vi "GetSingleAxisPos.vi"(6 "milliseconds to wait":u32=2, 8 "error in":errorcluster, 11 "Axis":T1={"System #"=0, "Axis ID"="", "Multiplier"=1.0}) -> (0 "error out":errorcluster, 3 "Position":dbl)   [LabVIEW 2011]
uses:
  PI_Axis.ctl
  PIAxisInfoGlobal.vi
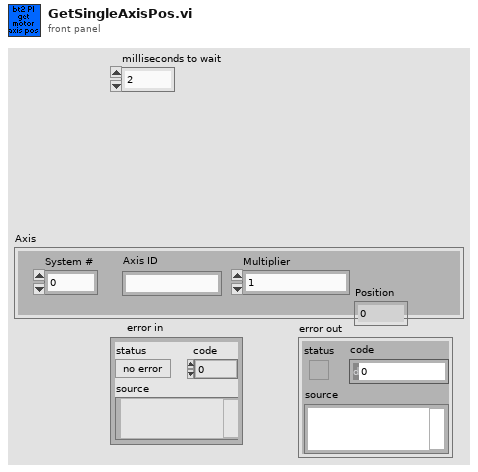
[diagram p1: front panel]
types:
  T1 = typedef "PI_Axis.ctl" = cluster{"System #":i32, "Axis ID":string, "Multiplier":dbl}
  T2 = typedef "GCS_Interface.ctl" = cluster{"MOV":refnum<vi>, "VEL":refnum<vi>, "VEL?":refnum<vi>, "POS?":refnum<vi>, "TMX?":refnum<vi>, "#7 (Ready?)":refnum<vi>, "FPL":refnum<vi>, "FNL":refnum<vi>}
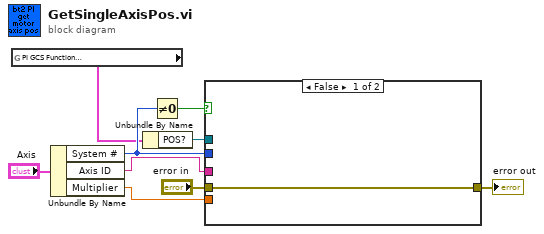
[diagram p0: block diagram]
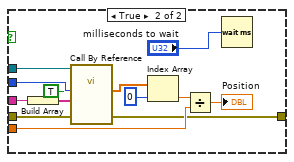
[diagram p2: hidden frame]
diagram:
  n1 = global read "PIAxisInfoGlobal.vi" "PI GCS Function\nReferences"() -> (w1:T2)
  n2 = Unbundle By Name("Axis") -> ("System #"=w7:i32, "Axis ID"=w8:string, "Multiplier"=w3:dbl)
  n3 = Unbundle By Name(w1) -> ("POS?"=w2:refnum<vi>)
  n4 = Not Equal To 0?(x=w7) -> (x != 0?=w6:bool)
  n5 = case shown="False" w6 {
    tunnel: w7 -> [_ w16]
    tunnel: w8 -> [_ w23]
    tunnel: "error in" -> [w10 w14]
    tunnel: [w10 w13] -> w4
    tunnel: w3 -> [_ w19]
    tunnel: w2 -> [_ w18]
    frame False {
    }
    frame True {
      n6 = Build Array(w23) -> (w17:string[])
      n7 = call-by-ref "?"(reference=w18, "System no."=w16, "Axes to query"=w17, "Axis identifier?"=TRUE, "error in"=w14) -> ("Position"=w15:dbl[], "error out"=w13:errorcluster)  [unwired: 15 in, 2 out]
      n8 = Index Array(array=w15, index=0) -> (element=w21:dbl)
      n9 = Divide(x=w21, y=w19) -> (x/y=→"Position":dbl)
      n10 = Wait (ms)(milliseconds to wait="milliseconds to wait") -> ()  [unwired: 1 out]
    }
  }
  "error out" <- w4
